vi "startup.vi"() -> ()   [LabVIEW 2022 SP3]
doc: "____\nHAMPEL SOFTWARE ENGINEERING v2.6.0 (2023-12-19 10:54)"
uses:
  Project/PROJECT_StartupSteps.ctl
  Libraries/hse-libraries/Source/hse-ui/Screens/Screen_Event.ctl
  Libraries/hse-libraries/Source/hse-application/hse-application.lvclass/hse-application.ctl
  Libraries/hse-libraries/Source/hse-dqmh/Controls/Module Display Scenarios.ctl
  a3842642-d9f2-4b31-9a04-9778e2d39186.vi
  Libraries/hse-libraries/Source/hse-application/HSE Application not initialized--error.vi
  Project/PROJECT_SplashScreen.vi
  Libraries/hse-libraries/Source/hse-application/hse-application__GetSingleton.vi
  <vilib>/Utility/sysdir.llb/Get System Directory.vi
  <vilib>/Utility/error.llb/Error Cluster From Error Code.vi
  Libraries/hse-libraries/Source/hse-configuration/config-ini/config-ini.lvclass
  Libraries/hse-libraries/Source/hse-ui/hse-ui.lvlib
  Project/Project.lvlib
  Libraries/hse-libraries/Source/hse-application/hse-application.lvclass
  Libraries/hse-libraries/Source/hse-dqmh/hse-dqmh-dynamicrequesters.lvlib
  <vilib>/Hampel Software Engineering/HSE Logger/hse-logger.lvlib
  Libraries/hse-libraries/Source/hse-dqmh/hse-dqmh.lvlib
  Libraries/hse-libraries/Source/hse-misc/hse-misc.lvlib
panel:
  out "Continue Startup UE":refnum<user-event>
  out "Modules List":path[](array[path])=[path "Modules/DB_CONNECTOR", path "Modules/S7com", path "Modules/VISU", path "Modules/LIVE-VIEW", path "Modules/SPH-ADMIN"]
  out "Start Module":string="SPH-ADMIN"
  # "Press the Run arrow to call the splash screen\nwhich waits for the actual application to start"
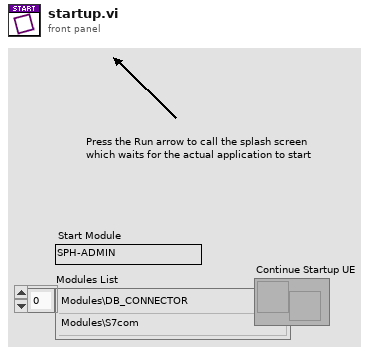
[diagram p1: front panel]
types:
  T1 = typedef "Project.lvlib/PROJECT_StartupSteps.ctl" = enum16{"Init", "Init Continue Startup", "Create Splash Event", "Open Splash VI", "Read Config File", "Wait for Continue Event", "Load Event Manager (static)", "Load UI Manager (static)", "Register for UI Status Event", "Load Modules (dynamic)", "Register Modules in UI", "Register Modules in EVH", "Set Runtime Menu in UI", "Configure statically loaded modules", "Set CLI Arguments", "Configure Modules", "Display Module in UI Subpanel", "Show UI Frontpanel", "Close Splash VI", "Wait for UI to quit", "Stop Modules", "Close Startup VI", "Error"}
  T2 = enum32{"Invalid", "Standard", "Closed", "Hidden", "Minimized", "Maximized"}
  T3 = typedef "hse-dqmh.lvlib/Module Display Scenarios.ctl" = enum16{"Stand-Alone", "Managed"}
  T4 = typedef "hse-ui.lvlib/Screen_Event.ctl" = cluster{"text":string, "percent":i32}
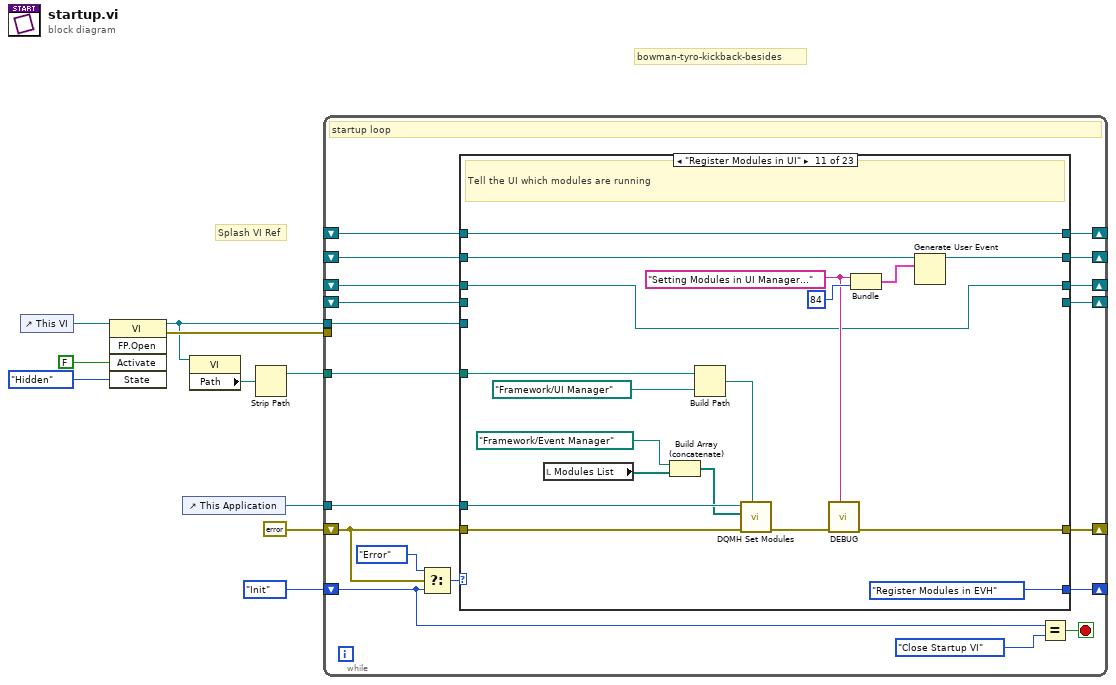
[diagram p0: block diagram]
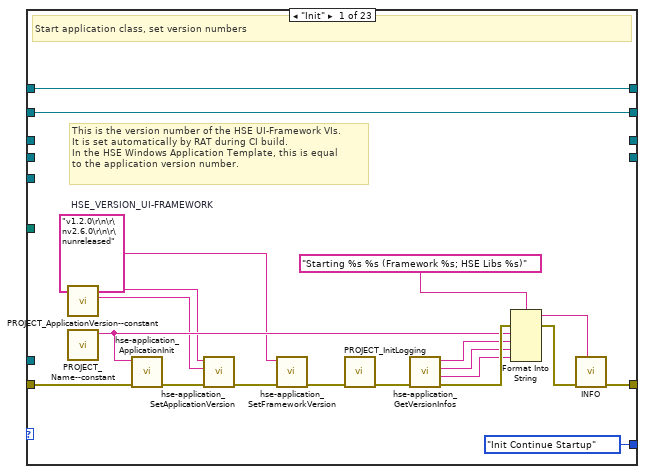
[diagram p2: hidden frame]
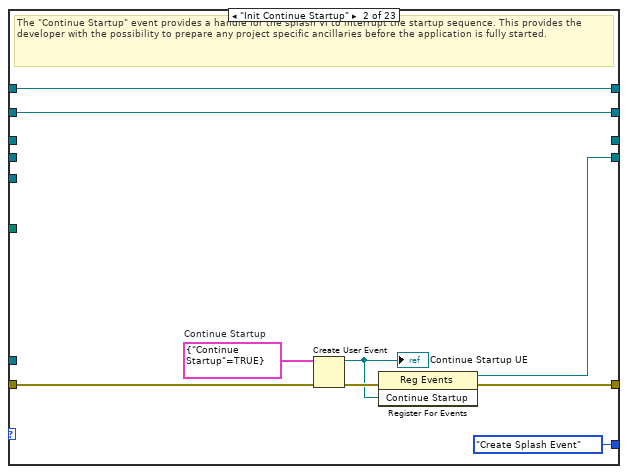
[diagram p3: hidden frame]
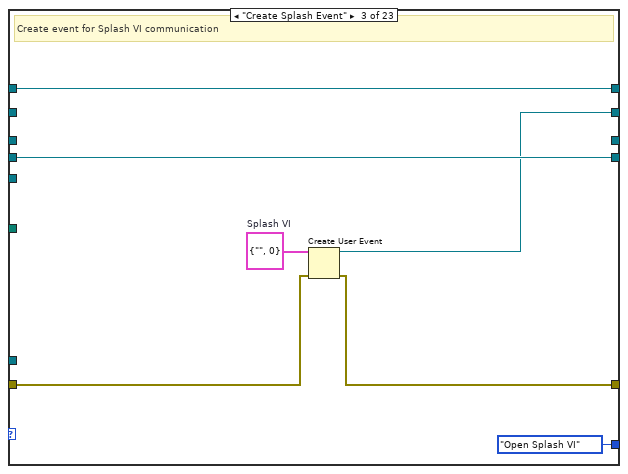
[diagram p4: hidden frame]
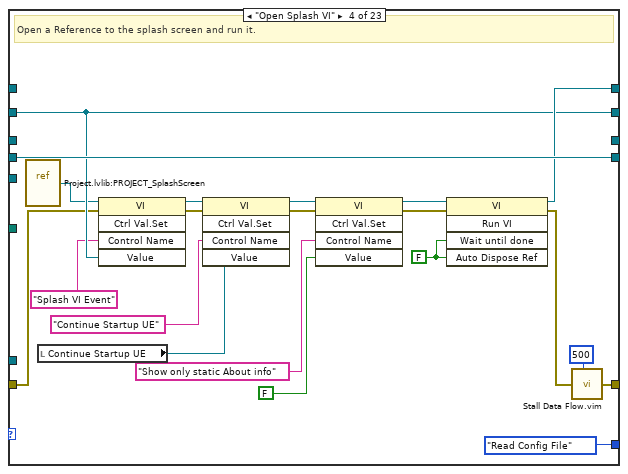
[diagram p5: hidden frame]
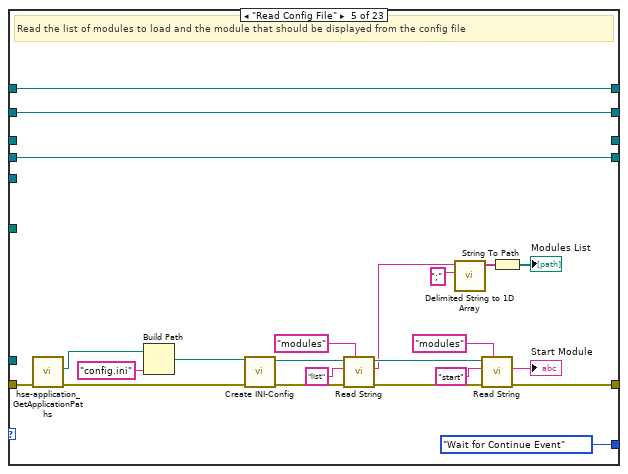
[diagram p6: hidden frame]
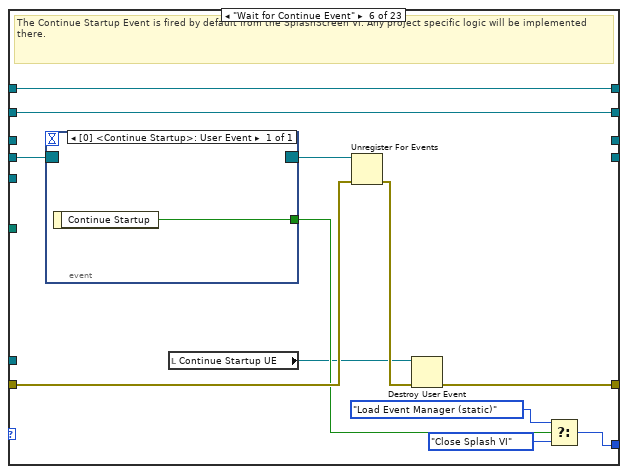
[diagram p7: hidden frame]
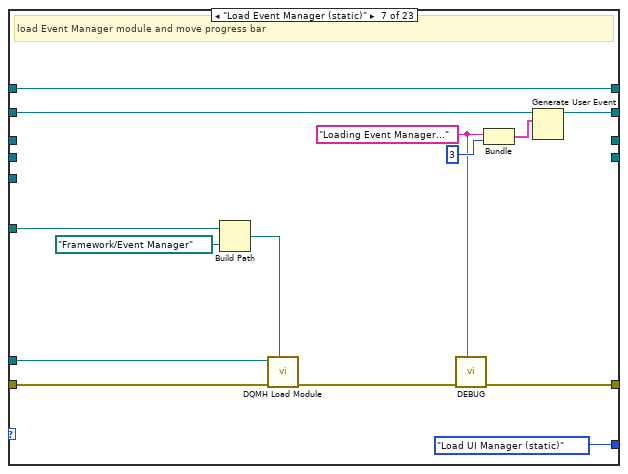
[diagram p8: hidden frame]
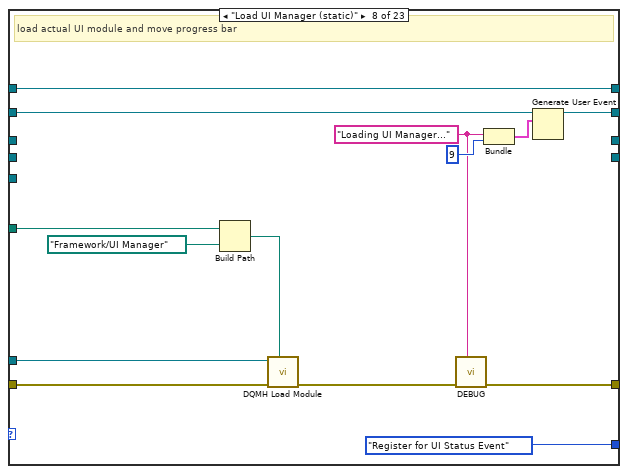
[diagram p9: hidden frame]
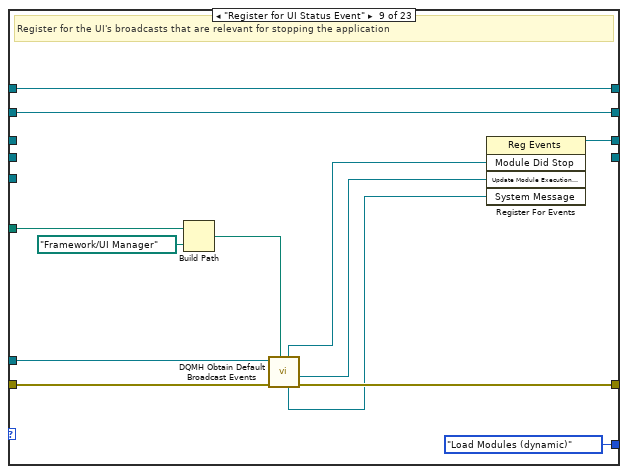
[diagram p10: hidden frame]
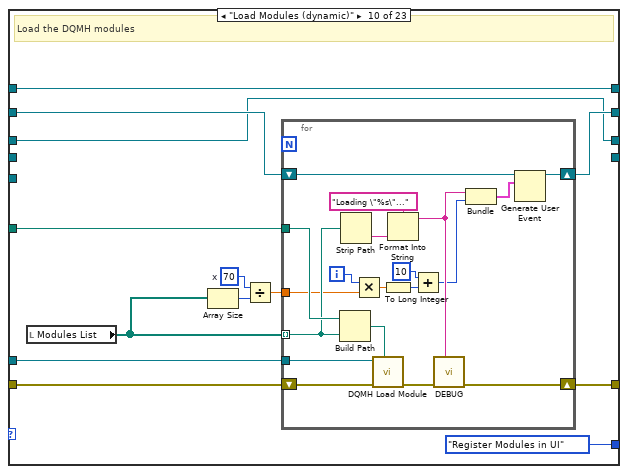
[diagram p11: hidden frame]
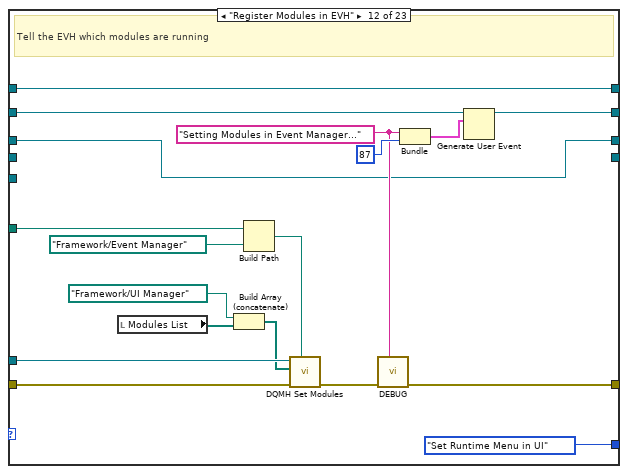
[diagram p12: hidden frame]
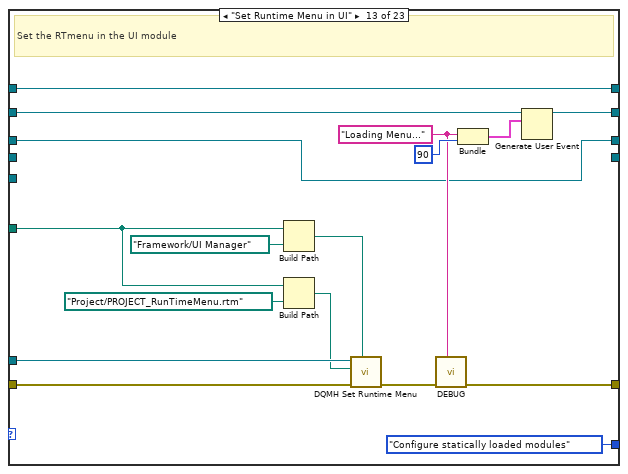
[diagram p13: hidden frame]
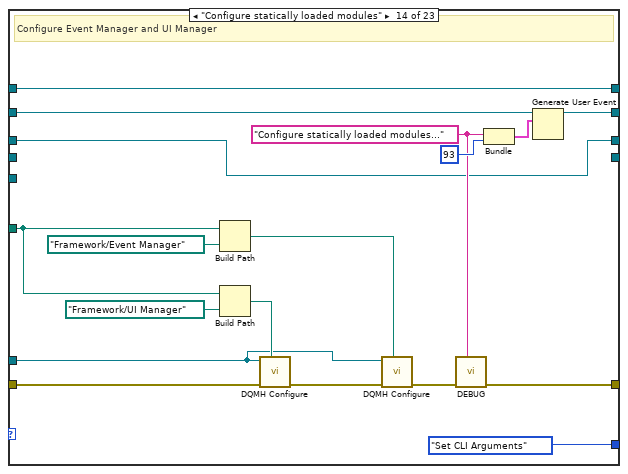
[diagram p14: hidden frame]
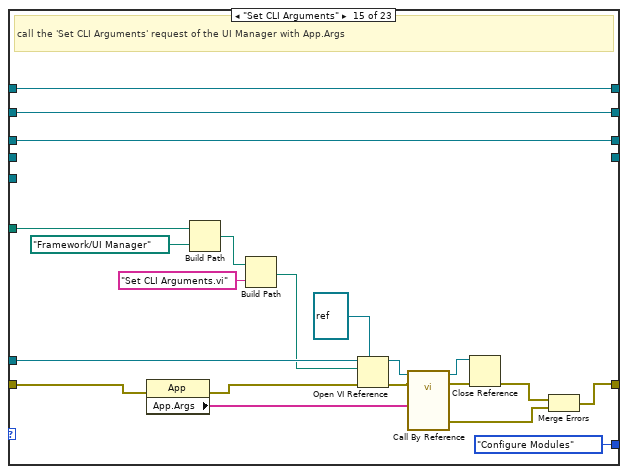
[diagram p15: hidden frame]
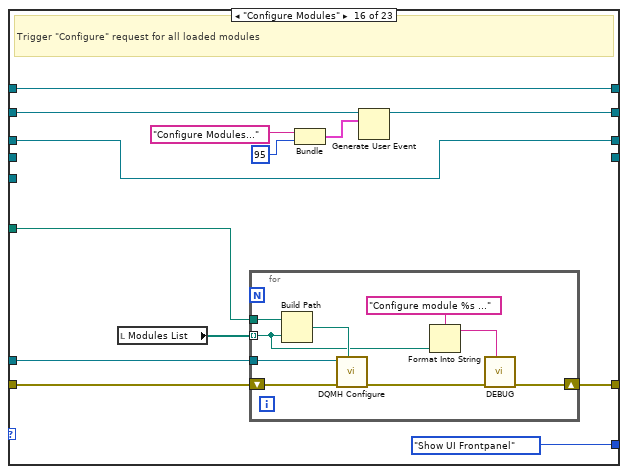
[diagram p16: hidden frame]
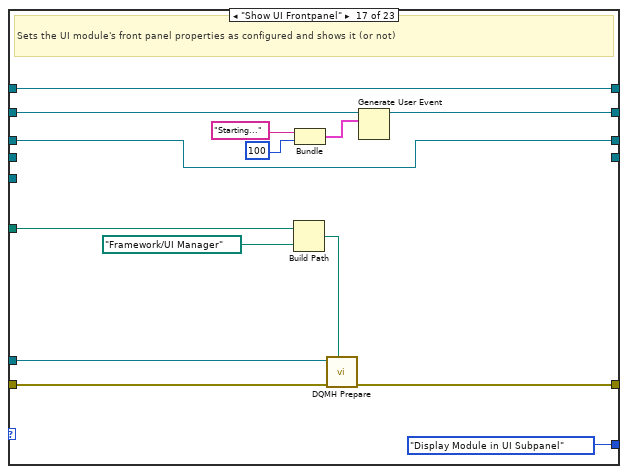
[diagram p17: hidden frame]
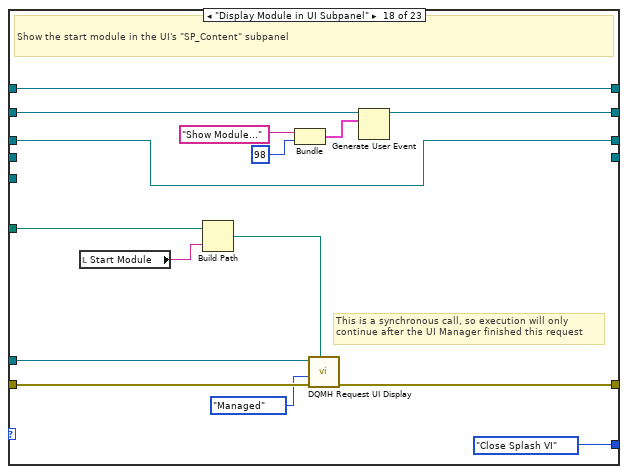
[diagram p18: hidden frame]
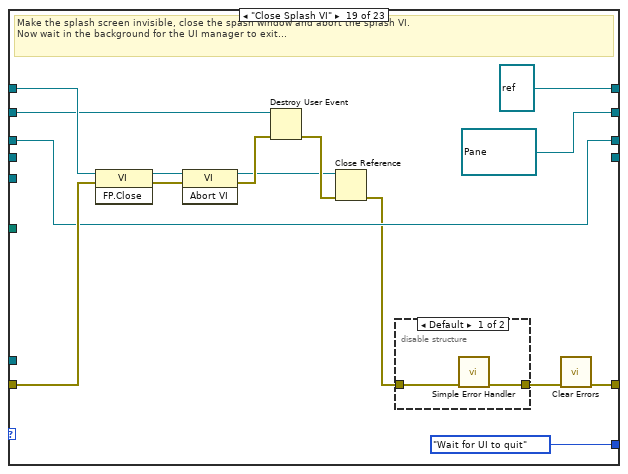
[diagram p19: hidden frame]
diagram:
  # "bowman-tyro-kickback-besides"
  # "Splash VI Ref"
  n1 = control-ref of="This VI"() -> (w7:refnum<vi>)
  n2 = invoke class="VI" method="FP.Open"(reference=w7, "Activate"=FALSE ("Activate?"), "State"=T2."Hidden") -> (reference out=w4:refnum<vi>, error out=w5:errorcluster)  [unwired: 2 in, 3 out]
  n3 = control-ref of="This Application"() -> (w1:refnum<vi>)
  n4 = property class="VI"(reference=w4) -> ("Path"=w3:path)  [unwired: 1 in, 2 out]
  n5 = Strip Path(path=w3) -> (stripped path=w2:path)  [unwired: 1 out]
  n6 = while {
    shift-right: [w27] -> _
    shift-left: errorcluster {"status"=FALSE, "code"=0, "source"=""} ("error out") -> [w22]
    shift-right: [w29] -> _
    shift-left: _ -> [w28]
    tunnel: w4 -> [w26]
    shift-right: [w25] -> _
    shift-left: _ -> [w24]
    shift-right: [w23] -> _
    shift-left: PROJECT_StartupSteps."Init" ("Startup Steps") -> [w19]
    tunnel: w5 -> [_]
    shift-right: [w16] -> _
    shift-left: _ -> [w15]
    tunnel: w2 -> [w14]
    tunnel: w1 -> [w13]
    shift-right: [w12] -> _
    shift-left: _ -> [w11]
    stop <- w17 stop-if-true
    # "startup loop"
    n7 = Select(t=PROJECT_StartupSteps."Error" ("Startup Steps"), s=w22, f=w19) -> (s? t:f=w21:T1)
    n8 = case shown="\"Register Modules in UI\"" w21 {
      selector: w21 -> [_ _ _ _ _ _ _ _ _ _ _ _ _ _ _ _ _ _ _ _ _ w415 _]
      tunnel: [w48 w50 w64 w85 w109 w114 w136 w150 w162 w176 w213 w231 w248 w266 w287 w300 w323 w338 refnum<vi> refnum w362 w395 _ refnum<vi> refnum] -> w29
      tunnel: w28 -> [w48 w50 w64 _ w109 w114 w136 w150 w162 w176 w213 w231 w248 w266 w287 w300 w323 w338 w351 w362 w395 _ w433]
      tunnel: w22 -> [w43 w58 w63 w81 w106 w121 w130 w144 w155 w174 w212 w230 w247 w261 w273 w291 w313 w337 w347 w359 w390 w414 w428]
      tunnel: [w38 w56 w62 w67 w97 w111 w126 w140 w154 w173 w201 w219 w237 w258 w268 w290 w315 w328 w348 w359 w392 w409 w431] -> w27
      tunnel: w26 -> [_ _ _ _ _ _ _ _ _ _ _ _ _ _ _ _ _ _ _ _ _ w416 _]
      tunnel: [w47 w51 w60 w83 w108 w113 w134 w148 w161 w171 w209 w227 w245 w264 w286 w295 w318 w332 refnum<user-event> refnum ("Splash VI") w361 w394 _ refnum<user-event> refnum ("Splash VI")] -> w25
      tunnel: w24 -> [w47 w51 _ w83 w108 w113 w135 w149 w161 w172 w210 w228 w246 w265 w286 w296 w319 w333 w350 w361 w394 _ w434]
      tunnel: [PROJECT_StartupSteps."Init Continue Startup" ("Startup Steps") PROJECT_StartupSteps."Create Splash Event" ("Startup Steps") PROJECT_StartupSteps."Open Splash VI" ("Startup Steps") PROJECT_StartupSteps."Read Config File" ("Startup Steps") PROJECT_StartupSteps."Wait for Continue Event" ("Startup Steps") w119 PROJECT_StartupSteps."Load UI Manager (static)" ("Startup Steps") PROJECT_StartupSteps."Register for UI Status Event" ("Startup Steps") PROJECT_StartupSteps."Load Modules (dynamic)" ("Startup Steps") PROJECT_StartupSteps."Register Modules in UI" ("Startup Steps") PROJECT_StartupSteps."Register Modules in EVH" ("Startup Steps") PROJECT_StartupSteps."Set Runtime Menu in UI" ("Startup Steps") PROJECT_StartupSteps."Configure statically loaded modules" ("Startup Steps") PROJECT_StartupSteps."Set CLI Arguments" ("Startup Steps") PROJECT_StartupSteps."Configure Modules" ("Startup Steps") PROJECT_StartupSteps."Show UI Frontpanel" ("Startup Steps") PROJECT_StartupSteps."Display Module in UI Subpanel" ("Startup Steps") PROJECT_StartupSteps."Close Splash VI" ("Startup Steps") PROJECT_StartupSteps."Wait for UI to quit" ("Startup Steps") w360 PROJECT_StartupSteps."Close Startup VI" ("Startup Steps") w415 PROJECT_StartupSteps."Stop Modules" ("Startup Steps")] -> w23
      tunnel: [_ _ _ _ _ _ _ _ w160 w164 w196 w214 w232 w249 w267 w288 w310 w324 w346 w357 _ _ _] -> w16
      tunnel: w15 -> [_ _ _ _ _ _ _ _ _ w164 w196 w214 w232 w249 w267 w288 w310 w324 w346 w358 w391 _ _]
      tunnel: w14 -> [_ _ _ _ _ _ w132 w146 w159 w170 w206 w224 w241 w252 w284 w293 w311 w330 _ _ w386 _ _]
      tunnel: w13 -> [_ _ _ _ _ _ w128 w142 w153 w169 w207 w225 w244 w250 w280 w289 w312 w329 _ _ w387 _ _]
      tunnel: [_ w52 w65 w86 w90 _ _ _ _ _ _ _ _ _ _ _ _ _ _ _ _ _ _] -> w12
      tunnel: w11 -> [_ _ w65 w86 w90 w120 _ _ _ _ _ _ _ _ _ _ _ _ _ _ _ _ _]
      frame "Init" {
        w30 = "v1.2.0\r\n\r\nv2.6.0\r\n\r\nunreleased"  # HSE_VERSION_UI-FRAMEWORK
        # "This is the version number of the HSE UI-Framework VIs.\nIt is set automatically by RAT during CI build.\nIn the HSE Windows Application Template, this is equal\nto the application version number."
        # "Start application class, set version numbers"
        n9 = call "PROJECT_ApplicationVersion--constant.vi"() -> ("HSE_VERSION_HISTORY"=w35:string, "HSE_VERSION_NUMBER"=w36:string)  [unwired: 10 in]
        n10 = call "PROJECT_Name--constant.vi"() -> ("PROJECT Name"=w40:string)  [unwired: 11 in]
        n11 = call "hse-application_ApplicationInit.vi"("error in"=w43, "Project Name"=w40) -> ("error out"=w46:errorcluster)  [unwired: 9 in]
        n12 = call "hse-application_SetApplicationVersion.vi"("error in"=w46, "Application Version History"=w35, "Application Version Number"=w36) -> ("error out"=w45:errorcluster)  [unwired: 8 in]
        n13 = call "hse-application_SetFrameworkVersion.vi"("error in"=w45, "Framework Version Number"=w30) -> ("error out"=w42:errorcluster)  [unwired: 9 in]
        n14 = call "PROJECT_InitLogging.vi"("error in"=w42) -> ("error out"=w34:errorcluster)  [unwired: 10 in]
        n15 = call "hse-application_GetVersionInfos.vi"("error in"=w34) -> ("error out"=w49:errorcluster, "HSE-LIB Version"=w33:string, "Framework Version"=w31:string, "Application Version"=w32:string)  [unwired: 5 in, 2 out]
        n16 = Format Into String(format string="Starting %s %s (Framework %s; HSE Libs %s)", error in=w49, w40, w32, w31, w33) -> (resulting string=w37:string, error out=w39:errorcluster)  [unwired: 1 in]
        n17 = call <vilib>:"INFO.vi"("Message"=w37, "error in"=w39) -> ("error out"=w38:errorcluster)  [unwired: 9 in]
      }
      frame "Init Continue Startup" {
        w54 = cluster{"Continue Startup":bool} {"Continue Startup"=TRUE}  # Continue Startup
        # "The \"Continue Startup\" event provides a handle for the splash VI to interrupt the startup sequence. This provides the developer with the possibility to prepare any project specific ancillaries before the application is fully started."
        n18 = Create User Event(user event datatype=w54, error in=w58) -> (user event=w55:refnum<user-event>, error out=w57:errorcluster)
        "Continue Startup UE" <- w55
        n19 = register-events(error in=w57, w55) -> (reference out=w52:refnum<event-registration>, error out=w56:errorcluster)  [unwired: 1 in]
      }
      frame "Create Splash Event" {
        w61 = T4 {"text"="", "percent"=0}  # Splash VI
        # "Create event for Splash VI communication"
        n20 = Create User Event(user event datatype=w61, error in=w63) -> (user event=w60:refnum<user-event>, error out=w62:errorcluster)
      }
      frame "Open Splash VI" {
        w84 = FALSE ("Wait Until Done")
        # "Open a Reference to the splash screen and run it."
        n21 = vi-ref "Project.lvlib:PROJECT_SplashScreen.vi"() -> (w69:refnum<vi>)
        n22 = local read "Continue Startup UE"() -> (w75:refnum<user-event>)
        n23 = invoke class="VI" method="Ctrl Val.Set"(reference=w69, error in=w81, "Control Name"="Splash VI Event", "Value"=w83) -> (reference out=w73:refnum<vi>, error out=w71:errorcluster)  [unwired: 1 in, 3 out]
        n24 = invoke class="VI" method="Ctrl Val.Set"(reference=w73, error in=w71, "Control Name"="Continue Startup UE", "Value"=w75) -> (reference out=w72:refnum<vi>, error out=w70:errorcluster)  [unwired: 1 in, 3 out]
        n25 = invoke class="VI" method="Ctrl Val.Set"(reference=w72, error in=w70, "Control Name"="Show only static About info", "Value"=FALSE ("Wait Until Done")) -> (reference out=w79:refnum<vi>, error out=w78:errorcluster)  [unwired: 1 in, 3 out]
        n26 = invoke class="VI" method="Run VI"(reference=w79, error in=w78, "Wait until done"=w84, "Auto Dispose Ref"=w84) -> (reference out=w85:refnum<vi>, error out=w68:errorcluster)  [unwired: 1 in, 3 out]
        n27 = call "Stall Data Flow.vim"("value in"=w68, "milliseconds to wait"=u32 500) -> ("value out"=w67:errorcluster)  [unwired: 1 out]
      }
      frame "Read Config File" {
        # "Read the list of modules to load and the module that should be displayed from the config file"
        n28 = call "hse-application_GetApplicationPaths.vi"("error in"=w106) -> ("error out"=w95:errorcluster, "Config Directory"=w103:path)  [unwired: 4 in, 5 out]
        n29 = Build Path(base path=w103, name or relative path="config.ini" ("format string")) -> (appended path=w96:path)
        n30 = call "Create INI-Config.vi"("error in"=w95, "INI Filepath"=w96) -> ("error out"=w94:errorcluster, "config-ini out"=w93:refnum<class "config-ini.lvclass">)  [unwired: 8 in]
        n31 = call-dynamic "Read String.vi"("Section"="modules", "error in"=w94, "Key"="list", "config-base in"=w93) -> ("error out"=w98:errorcluster, "Value"=w89:string, "config-base out"=w101:refnum<class "config-ini.lvclass">)  [unwired: 5 in]
        n32 = call "Delimited String to 1D Array.vi"("Delimiter (,)"=";" ("delimiter (Tab)"), "Delimited String"=w89) -> ("String Array"=w88:string[])  [unwired: 9 in]
        n33 = call-dynamic "Read String.vi"("Section"="modules", "error in"=w98, "Key"="start", "config-base in"=w101) -> ("error out"=w97:errorcluster, "Value"=→"Start Module":string)  [unwired: 5 in, 1 out]
        n34 = String To Path(string=w88) -> (path=→"Modules List":path[])
      }
      frame "Wait for Continue Event" {
        # "The Continue Startup Event is fired by default from the SplashScreen VI. Any project specific logic will be implemented there."
        n35 = event shown="[0] <Continue Startup>: User Event" {
          selector: w120 -> [_]
          dyn-events: [_] -> w115
          timeout: _ -> [_]
          tunnel: [w122] -> w116
          event User Event {
            n36 = event-data() -> ("Continue Startup"=w122:bool)  [unwired: 1 in]
          }
        }
        n37 = local read "Continue Startup UE"() -> (w110:refnum<user-event>)
        n38 = Unregister For Events(event registration refnum=w115, error in=w121) -> (error out=w112:errorcluster)
        n39 = Destroy User Event(user event=w110, error in=w112) -> (error out=w111:errorcluster)
        n40 = Select(t=PROJECT_StartupSteps."Load Event Manager (static)" ("Startup Steps"), s=w116, f=PROJECT_StartupSteps."Close Splash VI") -> (s? t:f=w119:T1)
      }
      frame "Load Event Manager (static)" {
        w123 = "Loading Event Manager..." ("text")
        # "load Event Manager module and move progress bar"
        n41 = Build Path(base path=w132, name or relative path=path "Framework/Event Manager") -> (appended path=w127:path)
        n42 = call "DQMH Load Module.vi"("Module Disk Path"=w127, "error in (no error)"=w130, "Application reference"=w128) -> ("error out"=w129:errorcluster)  [unwired: 8 in]
        n43 = call <vilib>:"DEBUG.vi"("Message"=w123, "error in"=w129) -> ("error out"=w126:errorcluster)  [unwired: 9 in]
        n44 = Bundle("text"=w123, 3) -> (w124:cluster{"text":string, i32})  [unwired: 1 in]
        n45 = Generate User Event(user event=w135, event data cluster=w124) -> (user event out=w134:refnum<user-event>)  [unwired: 2 in, 1 out]
      }
      frame "Load UI Manager (static)" {
        w137 = "Loading UI Manager..." ("text")
        # "load actual UI module and move progress bar"
        n46 = Build Path(base path=w146, name or relative path=path "Framework/UI Manager") -> (appended path=w141:path)
        n47 = call "DQMH Load Module.vi"("Module Disk Path"=w141, "error in (no error)"=w144, "Application reference"=w142) -> ("error out"=w143:errorcluster)  [unwired: 8 in]
        n48 = call <vilib>:"DEBUG.vi"("Message"=w137, "error in"=w143) -> ("error out"=w140:errorcluster)  [unwired: 9 in]
        n49 = Bundle("text"=w137, 9) -> (w138:cluster{"text":string, i32})  [unwired: 1 in]
        n50 = Generate User Event(user event=w149, event data cluster=w138) -> (user event out=w148:refnum<user-event>)  [unwired: 2 in, 1 out]
      }
      frame "Register for UI Status Event" {
        # "Register for the UI's broadcasts that are relevant for stopping the application"
        n51 = Build Path(base path=w159, name or relative path=path "Framework/UI Manager") -> (appended path=w157:path)
        n52 = call "DQMH Obtain Default Broadcast Events.vi"("Module Disk Path"=w157, "error in (no error)"=w155, "Application reference"=w153) -> ("error out"=w154:errorcluster, "Update Module Execution Status"=w156:refnum<user-event>, "System Message"=w151:refnum<user-event>, "Module Did Stop"=w152:refnum<user-event>)  [unwired: 3 in, 2 out]
        n53 = register-events(w152, w156, w151) -> (reference out=w160:refnum<event-registration>)  [unwired: 2 in, 1 out]
      }
      frame "Load Modules (dynamic)" {
        w167 = 70  # x
        # "Load the DQMH modules"
        n54 = local read "Modules List"() -> (w165:path[])
        n55 = Array Size(array=w165) -> (size(s)=w168:i32)
        n56 = Divide(x=w167, y=w168) -> (x/y=w166:dbl)
        n57 = for {
          tunnel: w165 -> [w189] mode=indexing
          shift-right: [w184] -> w173
          shift-left: w174 -> [w188]
          shift-right: [w194] -> w171
          shift-left: w172 -> [w195]
          tunnel: w170 -> [w190]
          tunnel: w169 -> [w186]
          tunnel: w166 -> [w183]
          i -> [w191]
          n58 = Build Path(base path=w190, name or relative path=w189) -> (appended path=w187:path)
          n59 = Strip Path(path=w189) -> (name=w192:string)  [unwired: 1 out]
          n60 = Multiply(x=w191, y=w183) -> (x*y=w182:dbl)
          n61 = call "DQMH Load Module.vi"("Module Disk Path"=w187, "error in (no error)"=w188, "Application reference"=w186) -> ("error out"=w185:errorcluster)  [unwired: 8 in]
          n62 = To Long Integer(number=w182) -> (32bit integer=w181:i32)
          n63 = Format Into String(format string="Loading \"%s\"..." ("text"), w192) -> (resulting string=w179:string)  [unwired: 2 in, 1 out]
          n64 = Add(x=10, y=w181) -> (x+y=w178:i32)
          n65 = call <vilib>:"DEBUG.vi"("Message"=w179, "error in"=w185) -> ("error out"=w184:errorcluster)  [unwired: 9 in]
          n66 = Bundle(w179, w178) -> (w180:cluster{string, i32})  [unwired: 1 in]
          n67 = Generate User Event(user event=w195, event data cluster=w180) -> (user event out=w194:refnum<user-event>)  [unwired: 2 in, 1 out]
        }
      }
      frame "Register Modules in UI" {
        w199 = "Setting Modules in UI Manager..." ("text")
        # "Tell the UI which modules are running"
        n68 = local read "Modules List"() -> (w203:path[])
        n69 = Build Array (concatenate)(path "Framework/Event Manager", w203) -> (w198:path[])
        n70 = Build Path(base path=w206, name or relative path=path "Framework/UI Manager") -> (appended path=w204:path)
        n71 = call "DQMH Set Modules.vi"("Module Disk Path"=w204, "error in (no error)"=w212, "modules to load dynamically"=w198, "Application reference"=w207) -> ("error out"=w202:errorcluster)  [unwired: 7 in]
        n72 = call <vilib>:"DEBUG.vi"("Message"=w199, "error in"=w202) -> ("error out"=w201:errorcluster)  [unwired: 9 in]
        n73 = Bundle("text"=w199, "y"=84) -> (w200:cluster{"text":string, "y":i32})  [unwired: 1 in]
        n74 = Generate User Event(user event=w210, event data cluster=w200) -> (user event out=w209:refnum<user-event>)  [unwired: 2 in, 1 out]
      }
      frame "Register Modules in EVH" {
        w217 = "Setting Modules in Event Manager..." ("text")
        # "Tell the EVH which modules are running"
        n75 = local read "Modules List"() -> (w221:path[])
        n76 = Build Array (concatenate)(path "Framework/UI Manager", w221) -> (w216:path[])
        n77 = Build Path(base path=w224, name or relative path=path "Framework/Event Manager") -> (appended path=w222:path)
        n78 = call "DQMH Set Modules.vi"("Module Disk Path"=w222, "error in (no error)"=w230, "modules to load dynamically"=w216, "Application reference"=w225) -> ("error out"=w220:errorcluster)  [unwired: 7 in]
        n79 = call <vilib>:"DEBUG.vi"("Message"=w217, "error in"=w220) -> ("error out"=w219:errorcluster)  [unwired: 9 in]
        n80 = Bundle("text"=w217, "y"=87) -> (w218:cluster{"text":string, "y":i32})  [unwired: 1 in]
        n81 = Generate User Event(user event=w228, event data cluster=w218) -> (user event out=w227:refnum<user-event>)  [unwired: 2 in, 1 out]
      }
      frame "Set Runtime Menu in UI" {
        w234 = "Loading Menu..." ("text")
        # "Set the RTmenu in the UI module"
        n82 = Build Path(base path=w241, name or relative path=path "Framework/UI Manager") -> (appended path=w239:path)
        n83 = Build Path(base path=w241, name or relative path=path "Project/PROJECT_RunTimeMenu.rtm" ("vi path")) -> (appended path=w242:path)
        n84 = call "DQMH Set Runtime Menu.vi"("Module Disk Path"=w239, "error in (no error)"=w247, "Path to .rtm file"=w242, "Application reference"=w244) -> ("error out"=w238:errorcluster)  [unwired: 7 in]
        n85 = call <vilib>:"DEBUG.vi"("Message"=w234, "error in"=w238) -> ("error out"=w237:errorcluster)  [unwired: 9 in]
        n86 = Bundle("text"=w234, "y"=90) -> (w235:cluster{"text":string, "y":i32})  [unwired: 1 in]
        n87 = Generate User Event(user event=w246, event data cluster=w235) -> (user event out=w245:refnum<user-event>)  [unwired: 2 in, 1 out]
      }
      frame "Configure statically loaded modules" {
        w255 = "Configure statically loaded modules..." ("text")
        # "Configure Event Manager and UI Manager"
        n88 = Build Path(base path=w252, name or relative path=path "Framework/Event Manager") -> (appended path=w251:path)
        n89 = Build Path(base path=w252, name or relative path=path "Framework/UI Manager") -> (appended path=w260:path)
        n90 = call "DQMH Configure.vi"("Module Disk Path"=w260, "error in (no error)"=w261, "Application reference"=w250) -> ("error out"=w259:errorcluster)  [unwired: 8 in]
        n91 = call "DQMH Configure.vi"("Module Disk Path"=w251, "error in (no error)"=w259, "Application reference"=w250) -> ("error out"=w254:errorcluster)  [unwired: 8 in]
        n92 = call <vilib>:"DEBUG.vi"("Message"=w255, "error in"=w254) -> ("error out"=w258:errorcluster)  [unwired: 9 in]
        n93 = Bundle("text"=w255, 93) -> (w256:cluster{"text":string, i32})  [unwired: 1 in]
        n94 = Generate User Event(user event=w265, event data cluster=w256) -> (user event out=w264:refnum<user-event>)  [unwired: 2 in, 1 out]
      }
      frame "Set CLI Arguments" {
        # "call the 'Set CLI Arguments' request of the UI Manager with App.Args"
        n95 = property class="App"(error in=w273) -> (error out=w272:errorcluster, "App.Args"=w274:string[])  [unwired: 1 in, 1 out]
        n96 = Build Path(base path=w284, name or relative path=path "Framework/UI Manager") -> (appended path=w282:path)
        n97 = Build Path(base path=w282, name or relative path="Set CLI Arguments.vi") -> (appended path=w275:path)
        n98 = Open VI Reference(type specifier VI Refnum (for type only)=refnum<vi> refnum, application reference (local)=w280, vi path=w275, error in (no error)=w272) -> (vi reference=w278:refnum<vi>, error out=w279:errorcluster)  [unwired: 2 in]
        n99 = call-by-ref "?"(reference=w278, error in=w279, "CLI Arguments"=w274) -> (reference out=w276:refnum<vi>, error out=w277:errorcluster, 0:"error out"=w270:errorcluster)  [unwired: 9 in, 1 out]
        n100 = Close Reference(reference=w276, error in (no error)=w277) -> (error out=w269:errorcluster)
        n101 = Merge Errors(w269, w270) -> (w268:errorcluster)
      }
      frame "Configure Modules" {
        # "Trigger \"Configure\" request for all loaded modules"
        n102 = local read "Modules List"() -> (w292:path[])
        n103 = for {
          tunnel: w293 -> [w309]
          tunnel: w292 -> [w302] mode=indexing
          tunnel: w289 -> [w307]
          shift-right: [w304] -> w290
          shift-left: w291 -> [w308]
          n104 = Build Path(base path=w309, name or relative path=w302) -> (appended path=w306:path)
          n105 = call "DQMH Configure.vi"("Module Disk Path"=w306, "error in (no error)"=w308, "Application reference"=w307) -> ("error out"=w305:errorcluster)  [unwired: 8 in]
          n106 = Format Into String(format string="Configure module %s ...", w302) -> (resulting string=w301:string)  [unwired: 2 in, 1 out]
          n107 = call <vilib>:"DEBUG.vi"("Message"=w301, "error in"=w305) -> ("error out"=w304:errorcluster)  [unwired: 9 in]
        }
        n108 = Bundle("text"="Configure Modules...", "y"=95) -> (w299:cluster{"text":string, "y":i32})  [unwired: 1 in]
        n109 = Generate User Event(user event=w296, event data cluster=w299) -> (user event out=w295:refnum<user-event>)  [unwired: 2 in, 1 out]
      }
      frame "Show UI Frontpanel" {
        # "Sets the UI module's front panel properties as configured and shows it (or not)"
        n110 = Build Path(base path=w311, name or relative path=path "Framework/UI Manager") -> (appended path=w314:path)
        n111 = Bundle("text"="Starting...", "y"=100) -> (w322:cluster{"text":string, "y":i32})  [unwired: 1 in]
        n112 = call "DQMH Prepare.vi"("Module Disk Path"=w314, "error in (no error)"=w313, "Application reference"=w312) -> ("error out"=w315:errorcluster)  [unwired: 8 in]
        n113 = Generate User Event(user event=w319, event data cluster=w322) -> (user event out=w318:refnum<user-event>)  [unwired: 2 in, 1 out]
      }
      frame "Display Module in UI Subpanel" {
        # "This is a synchronous call, so execution will only \ncontinue after the UI Manager finished this request"
        # "Show the start module in the UI's \"SP_Content\" subpanel"
        n114 = local read "Start Module"() -> (w326:string)
        n115 = Build Path(base path=w330, name or relative path=w326) -> (appended path=w325:path)
        n116 = Bundle("text"="Show Module...", "y"=98) -> (w336:cluster{"text":string, "y":i32})  [unwired: 1 in]
        n117 = call "DQMH Request UI Display.vi"("Module DIsk Path"=w325, "error in (no error)"=w337, "Display Scenario"=Module_Display_Scenarios."Managed" ("Module Display Scenarios"), "Application reference"=w329) -> ("error out"=w328:errorcluster)  [unwired: 6 in, 1 out]
        n118 = Generate User Event(user event=w333, event data cluster=w336) -> (user event out=w332:refnum<user-event>)  [unwired: 2 in, 1 out]
      }
      frame "Close Splash VI" {
        # "Make the splash screen invisible, close the spash window and abort the splash VI. \nNow wait in the background for the UI manager to exit..."
        n119 = invoke class="VI" method="FP.Close"(reference=w351, error in=w347) -> (reference out=w353:refnum<vi>, error out=w352:errorcluster)  [unwired: 1 in, 1 out]
        n120 = invoke class="VI" method="Abort VI"(reference=w353, error in=w352) -> (reference out=w339:refnum<vi>, error out=w344:errorcluster)  [unwired: 1 in, 1 out]
        n121 = Destroy User Event(user event=w350, error in=w344) -> (error out=w341:errorcluster)
        n122 = Close Reference(reference=w339, error in (no error)=w341) -> (error out=w340:errorcluster)
        n123 = disable-structure shown="Default" {
          disable-tunnel: [w355 w356] -> w349
          disable-tunnel: w340 -> [w354 w356]
          frame condition #0 (active) {
            n124 = call <vilib>:"Simple Error Handler.vi"("error in (no error)"=w354) -> ("error out"=w355:errorcluster)  [unwired: 4 in, 4 out]
          }
          frame condition #1 {
          }
        }
        n125 = call <vilib>:"Clear Errors.vi"("error in (no error)"=w349) -> ("error out"=w348:errorcluster)  [unwired: 5 in, 1 out]
      }
      frame "Wait for UI to quit" {
        # "Wait for one of the broadcasts that signal that the UI module exits."
        n126 = event shown="[2] <System Message>: User Event" {
          selector: w358 -> [_ _ _]
          dyn-events: [_ _ _] -> w357
          timeout: _ -> [_ _ _]
          tunnel: [w363 PROJECT_StartupSteps."Stop Modules" ("Startup Steps") w369] -> w360
          event User Event {
            # "Stop if UI Manager state changes to \"not running\""
            n127 = event-data() -> ("Running?"=w366:bool)  [unwired: 1 in]
            n128 = Select(t=PROJECT_StartupSteps."Wait for UI to quit" ("Startup Steps"), s=w366, f=PROJECT_StartupSteps."Stop Modules" ("Startup Steps")) -> (s? t:f=w363:T1)
          }
          event User Event {
            # "stop if UI Manager broadcasts it is stopping"
            n129 = event-data() -> ()  [unwired: 1 in, 3 out]
          }
          event User Event {
            # "Stop if UI Manager broadcasts to shutdown the application.\nThis is the expected scenario!"
            n130 = event-data() -> ("Identifier"=w373:string)  [unwired: 1 in]
            n131 = Equal?(x=w373, y="Shutdown Application") -> (x = y?=w368:bool)
            n132 = Select(t=PROJECT_StartupSteps."Stop Modules" ("Startup Steps"), s=w368, f=PROJECT_StartupSteps."Wait for UI to quit" ("Startup Steps")) -> (s? t:f=w369:T1)
          }
        }
      }
      frame "Stop Modules" {
        # "completely ignore this \nerror as we might not\neven have registered yet"
        # "remove error so that\nlast case is definitely\n\"Close Startup VI\""
        # "Stop all modules in case of error or shutdown"
        n133 = local read "Modules List"() -> (w388:path[])
        n134 = Reverse 1D Array(array=w388) -> (reversed array=w374:path[])
        n135 = for {
          tunnel: w374 -> [w405] mode=indexing
          tunnel: [w408] -> w376 mode=indexing
          tunnel: w390 -> [_]
          tunnel: w386 -> [w406]
          shift-right: [w403] -> w375
          shift-left: w387 -> [w403]
          n136 = Build Path(base path=w406, name or relative path=w405) -> (appended path=w404:path)
          n137 = call "DQMH Stop Module.vi"("Module Disk Path"=w404, "error in (no error)"=errorcluster {"status"=FALSE, "code"=0, "source"=""}, "Application ref"=w403) -> ("error out"=w408:errorcluster)  [unwired: 8 in]
        }
        n138 = Build Path(base path=w386, name or relative path=path "Framework/Event Manager") -> (appended path=w381:path)
        n139 = Build Path(base path=w386, name or relative path=path "Framework/UI Manager") -> (appended path=w382:path)
        n140 = flat-sequence {
          tunnel: w382 -> [w398]
          tunnel: [w396] -> w380
          tunnel: [w397] -> w378
          tunnel: w375 -> [w396]
          tunnel: w381 -> [w402]
          tunnel: w380 -> [w401]
          tunnel: [w400] -> w379
          tunnel: w378 -> [w400]
          tunnel: [w399] -> w377
          frame #0 {
            n141 = call "DQMH Stop Module.vi"("Module Disk Path"=w398, "Application ref"=w396) -> ("error out"=w397:errorcluster)  [unwired: 9 in]
          }
          frame #1 {
            n142 = call "DQMH Stop Module.vi"("Module Disk Path"=w402, "Application ref"=w401) -> ("error out"=w399:errorcluster)  [unwired: 9 in]
          }
        }
        n143 = Unregister For Events(event registration refnum=w391) -> (error out=w383:errorcluster)  [unwired: 1 in]
        n144 = call <vilib>:"Clear Errors.vi"("error in (no error)"=w383) -> ()  [unwired: 5 in, 2 out]
        n145 = Merge Errors(w377, w379, w376) -> (w389:errorcluster)
        n146 = call <vilib>:"Clear Errors.vi"("error in (no error)"=w389) -> ("error out"=w392:errorcluster)  [unwired: 5 in, 1 out]
      }
      frame "Close Startup VI" {
        # "Close the FP of this VI"
        n147 = call <vilib>:"INFO.vi"("Message"="Application stopped.", "error in"=w414) -> ("error out"=w413:errorcluster)  [unwired: 9 in]
        n148 = call <vilib>:"Close Logging.vi"("error in"=w413) -> ("error out"=w412:errorcluster)  [unwired: 10 in]
        n149 = call "hse-application_ApplicationShutdown.vi"("error in"=w412) -> ("error out"=w410:errorcluster)  [unwired: 10 in]
        n150 = disable-structure shown="Default" {
          disable-tunnel: w416 -> [w419 _]
          disable-tunnel: w410 -> [w418 w420]
          disable-tunnel: [w417 w420] -> w409
          frame condition #0 (active) {
            # "When in Dev. Env."
            n151 = invoke class="VI" method="FP.Close"(reference=w419, error in=w418) -> (error out=w417:errorcluster)  [unwired: 1 in, 2 out]
          }
          frame condition #1 {
            w421 = TRUE  # quit? (T)
            n152 = Quit LabVIEW(quit? (T)=w421) -> ()
          }
        }
      }
      frame "Error" {
        n153 = Unbundle By Name(w428) -> ("source"=w425:string)
        n154 = invoke class="VI" method="FP.Close"(reference=w433) -> (reference out=w437:refnum<vi>, error out=w436:errorcluster)  [unwired: 2 in, 1 out]
        n155 = call "hse-application_GetApplicationPaths.vi"() -> ("Data Directory"=w423:path)  [unwired: 5 in, 6 out]
        n156 = Format Into String(format string="Error during startup!\n\n%s\n\nMore information might be available in the logs in the data directory\n%s", w425, w423) -> (resulting string=w424:string)  [unwired: 2 in, 1 out]
        n157 = invoke class="VI" method="Abort VI"(reference=w437, error in=w436) -> (reference out=w439:refnum<vi>, error out=w438:errorcluster)  [unwired: 1 in, 1 out]
        n158 = Bundle By Name(cluster=w428, "source"=w424) -> (w427:errorcluster)
        n159 = Close Reference(reference=w439, error in (no error)=w438) -> (error out=w435:errorcluster)
        n160 = call "Dialogue_Error.vi"("error in"=w427) -> ()  [unwired: 10 in, 1 out]
        n161 = call <vilib>:"ERROR.vi"("Message"="Error during App initialization.", "error in"=w428) -> ()  [unwired: 9 in, 1 out]
        n162 = Destroy User Event(user event=w434, error in=w435) -> (error out=w432:errorcluster)
        n163 = call <vilib>:"Clear Errors.vi"("error in (no error)"=w432) -> ("error out"=w431:errorcluster)  [unwired: 5 in, 1 out]
      }
    }
    n164 = Equal?(x=w19, y=PROJECT_StartupSteps."Close Startup VI" ("Startup Steps")) -> (x = y?=w17:bool)
  }
